vi "Ping_lights.vi"() -> ()   [LabVIEW 2012]
panel:
  out "cluster":T1
  in  "stop":bool
  # "BAXTER HEAD LIGHTS"
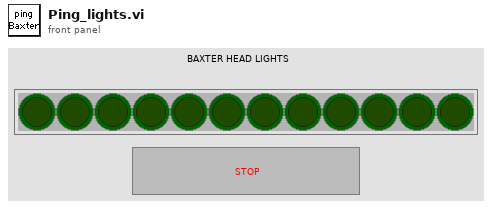
[diagram p1: front panel]
types:
  T1 = cluster{"[0]":bool, "[1]":bool, "[2]":bool, "[3]":bool, "[4]":bool, "[5]":bool, "[6]":bool, "[7]":bool, "[8]":bool, "[9]":bool, "[10]":bool, "[11]":bool}
  T2 = cluster{"Behavior":bool, "All On":bool, "All Off":bool, "Individual":bool[]}
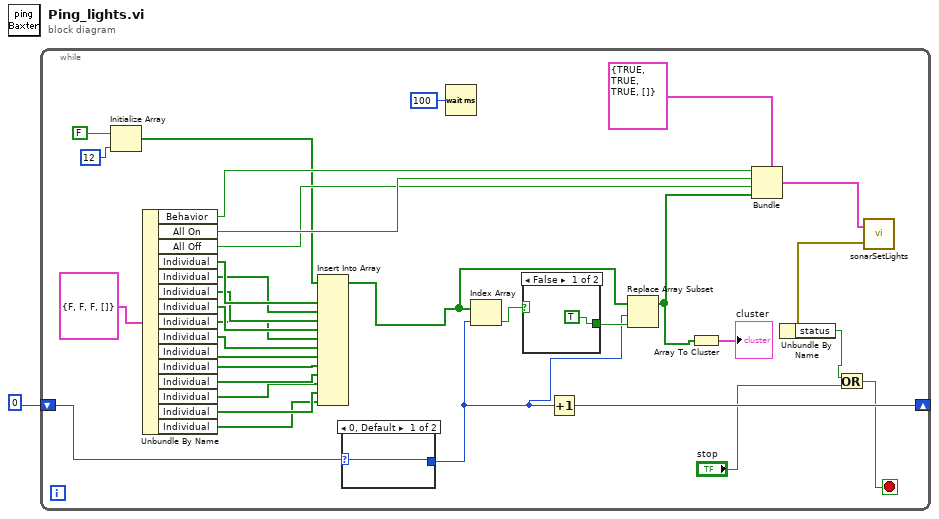
[diagram p0: block diagram]
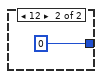
[diagram p2: hidden frame]
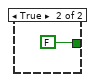
[diagram p3: hidden frame]
diagram:
  n1 = while {
    shift-right: [w13] -> _
    shift-left: 0 -> [w12]
    stop <- w7 stop-if-true
    n2 = Initialize Array(FALSE, 12 ("dimension size")) -> (w4:bool[])
    n3 = Unbundle By Name(T2 {"Behavior"=FALSE, "All On"=FALSE, "All Off"=FALSE, "Individual"=[]} ("Lights")) -> ("Behavior"=w19:bool, "All On"=w18:bool, "All Off"=w17:bool, "Individual"=w34:bool[], "Individual"=w33:bool[], "Individual"=w32:bool[], "Individual"=w31:bool[], "Individual"=w30:bool[], "Individual"=w29:bool[], "Individual"=w28:bool[], "Individual"=w27:bool[], "Individual"=w26:bool[], "Individual"=w25:bool[], "Individual"=w24:bool[], "Individual"=w23:bool[])
    n4 = Insert Into Array(array=w4, new element #1=w34, new element #2=w33, new element #3=w32, new element #4=w31, new element #5=w30, new element #6=w29, new element #7=w28, new element #8=w27, new element #9=w26, new element #10=w25, new element #11=w24, new element #12=w23) -> (w22:bool[])  [unwired: 1 in]
    n5 = case shown="0, Default" w12 {
      selector: w12 -> [w36 _]
      tunnel: [w36 0] -> w11
      frame 0, Default {
      }
      frame 12 {
      }
    }
    n6 = Wait (ms)(milliseconds to wait=u32 100) -> ()  [unwired: 1 out]
    n7 = Index Array(array=w22, index=w11) -> (element=w15:bool)
    n8 = case shown="False" w15 {
      tunnel: [TRUE FALSE] -> w14
      frame False {
      }
      frame True {
      }
    }
    n9 = Increment(x=w11) -> (x+1=w13:i32)
    n10 = Replace Array Subset(array=w22, new element=w14, index=w11) -> (w3:bool[])
    n11 = Array To Cluster(array=w3) -> (cluster=→"cluster":T1)
    n12 = Bundle(cluster=cluster{bool, bool, bool, bool[]} {TRUE, TRUE, TRUE, []}, w19, w18, w17, w3) -> (w20:cluster{bool, bool, bool, bool[]})
    n13 = call <userlib>:"sonarSetLights.vi"("Lights"=w20) -> ("error out"=w10:errorcluster)  [unwired: 3 in]
    n14 = Unbundle By Name(w10) -> ("status"=w9:bool)
    n15 = Or(x=w9, y="stop") -> (x .or. y?=w7:bool)
  }
